vi "CheckValidQueueReference.vi"(8 "error in":errorcluster, 11 "message ref in":refnum<class "CLM_LocalMessage_Queue.lvclass">) -> (0 "error out":errorcluster, 2 "valid?":bool, 3 "message ref out":refnum<class "CLM_LocalMessage_Queue.lvclass">)   [LabVIEW 2013, in "CLM_LocalMessage_Queue.lvclass"]
uses:
  CLM_LocalMessage_Queue.lvclass
  CLM_LocalMessage_Queue.lvclass/CLM_LocalMessage_Queue.ctl
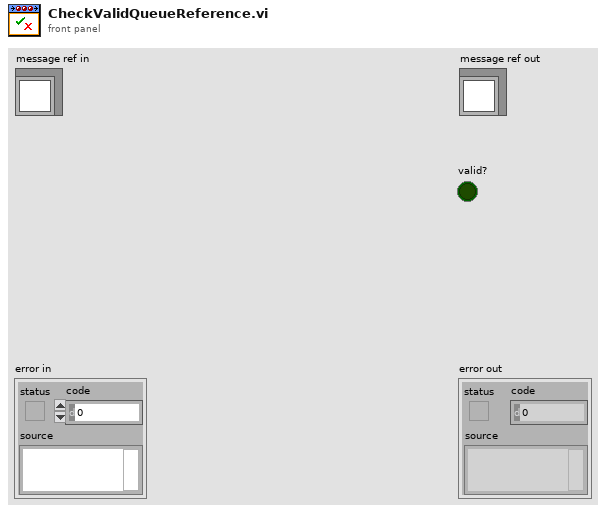
[diagram p1: front panel]
types:
  T1 = typedef "CLM_LocalMessage_Queue.lvclass/MessageQueue.ctl" = refnum<queue>
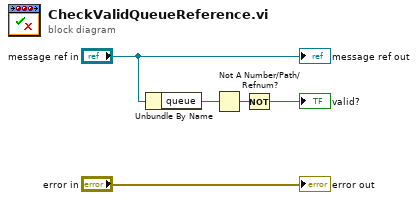
[diagram p0: block diagram]
diagram:
  n1 = Unbundle By Name("message ref in") -> ("queue"=w3:T1)
  n2 = Not A Number/Path/Refnum?(number/path/refnum=w3) -> (NaN/Path/Refnum?=w2:bool)
  n3 = Not(x=w2) -> (.not. x?=→"valid?":bool)
  "error out" <- "error in"
  "message ref out" <- "message ref in"
